vi "BoolToTrueFalse.vi"(1 "Boolean":bool) -> (0 "String":string)   [LabVIEW 2017, in "GPString.lvlib"]
doc: "Converts the <B>Boolean</B> input value to a \"True\" or \"False\" <B>String</B>.\n\nThis VI is inlined.\n\nSteen Schmidt\nGPower\n24/1 2013"
uses:
  GPString.lvlib
panel:
  # "Copyright © 2013\nSteen Schmidt, GPower\nSee enclosed license file for terms and conditions"
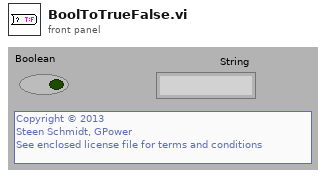
[diagram p1: front panel]
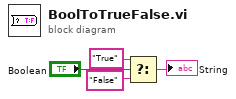
[diagram p0: block diagram]
diagram:
  n1 = Select(t="True", s="Boolean", f="False") -> (s? t:f=→"String":string)
